vi "set_ai_data_format.vi"(8 "error in (no error)":errorcluster, 10 "Data format":enum16{"Hexadecimal", "Engineering"}(ring), 11 "Modbus Master in":refnum<class "Modbus Master.lvclass">) -> (0 "error out":errorcluster, 3 "Modbus Master out":refnum<class "Modbus Master.lvclass">)   [LabVIEW 2018]
uses:
  <vilib>/NI/Modbus Library/API/Master/Modbus Master.lvclass
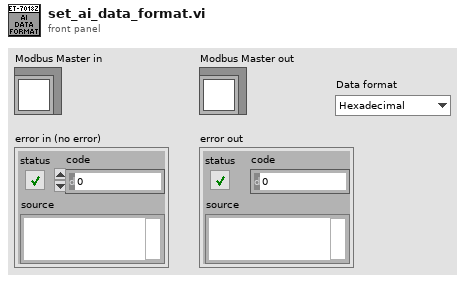
[diagram p1: front panel]
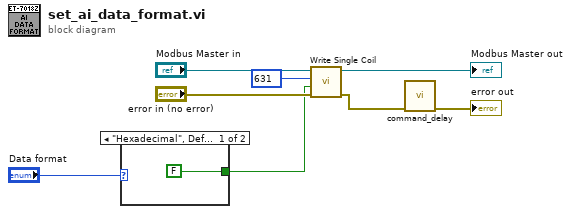
[diagram p0: block diagram]
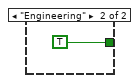
[diagram p2: hidden frame]
diagram:
  n1 = case shown="\"Hexadecimal\", Default" "Data format" {
    tunnel: [FALSE TRUE] -> w3
    frame "Hexadecimal", Default {
    }
    frame "Engineering" {
    }
  }
  n2 = call-dynamic "Write Single Coil.vi"("error in"="error in (no error)", "coil to write"=w3, "address"=u16 631 ("starting address"), "Modbus master in"="Modbus Master in") -> ("error out"=w2:errorcluster, "Modbus master out"=→"Modbus Master out":refnum<class "Modbus Master.lvclass">)  [unwired: 6 in]
  n3 = call "command_delay.vi"("error in (no error)"=w2) -> ("error out"=→"error out":errorcluster)  [unwired: 10 in]
